vi "Read.vi"(8 "error in (no error)":errorcluster, 11 "Add_WFM in":refnum<class "AbsFunc_Two Term_WFM_Numeric.lvclass">) -> (0 "error out":errorcluster, 2 "Waveform":waveform(dbl), 3 "Add_WFM out":refnum<class "AbsFunc_Two Term_WFM_Numeric.lvclass">)   [LabVIEW 2021, in "AbsFunc_Two Term_WFM_Numeric.lvclass"]
uses:
  AbsFunc_Two Term_WFM_Numeric.lvclass
  AbsFunc_Two Term_WFM_Numeric.lvclass/AbsFunc_Two Term_WFM_Numeric.ctl
  Abs_Types/Waveform/Abs_Waveform.lvclass
  Abs_Types/Numeric/Abs_Numeric.lvclass
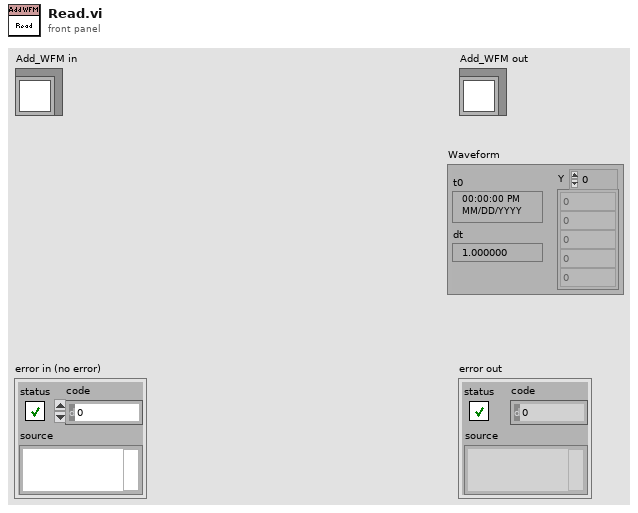
[diagram p1: front panel]
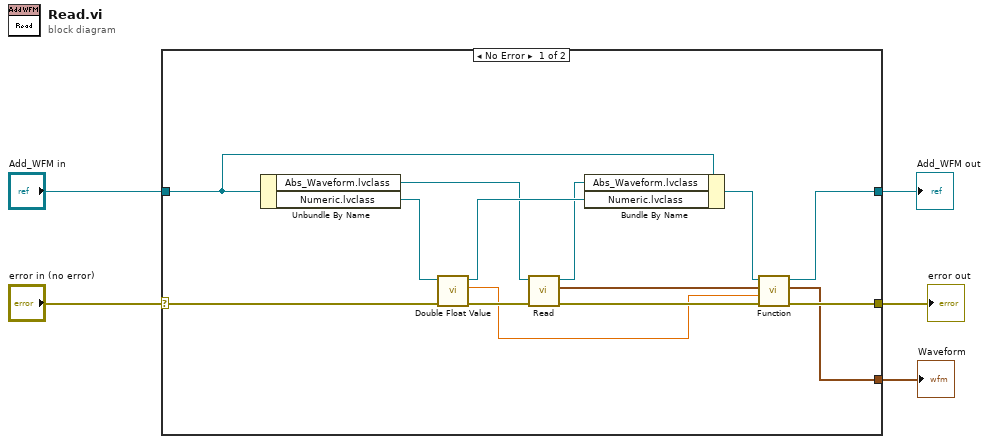
[diagram p0: block diagram]
diagram:
  n1 = case shown="No Error" "error in (no error)" {
    selector: "error in (no error)" -> [w18 w20]
    tunnel: [w19 w20] -> w5
    tunnel: [w16 w21] -> w4
    tunnel: "Add_WFM in" -> [w17 w21]
    tunnel: [w15 _] -> w1
    frame No Error {
      n2 = Unbundle By Name(w17) -> ("Abs_Waveform.lvclass"=w10:refnum<class "Abs_Waveform.lvclass">, "Numeric.lvclass"=w12:refnum<class "Abs_Numeric.lvclass">)
      n3 = call-dynamic "Double Float Value.vi"("error in (no error)"=w18, "Numeric in"=w12) -> ("error out"=w8:errorcluster, "Double"=w6:dbl, "Numeric out"=w11:refnum<class "Abs_Numeric.lvclass">)  [unwired: 7 in]
      n4 = call-dynamic "Read.vi"("error in (no error)"=w8, "Abs_Waveform in"=w10) -> ("error out"=w14:errorcluster, "Waveform"=w7:waveform(dbl), "Abs_Waveform out"=w9:refnum<class "Abs_Waveform.lvclass">)  [unwired: 7 in]
      n5 = Bundle By Name(cluster=w17, "Abs_Waveform.lvclass"=w9, "Numeric.lvclass"=w11) -> (w13:refnum<class "AbsFunc_Two Term_WFM_Numeric.lvclass">)
      n6 = call-dynamic "Function.vi"("error in (no error)"=w14, "Numeric"=w6, "Waveform"=w7, "Two Terminal in"=w13) -> ("error out"=w19:errorcluster, "Result"=w15:waveform(dbl), "Two Terminal out"=w16:refnum<class "AbsFunc_Two Term_WFM_Numeric.lvclass">)  [unwired: 5 in]
    }
    frame Error {
    }
  }
  "error out" <- w5
  "Add_WFM out" <- w4
  "Waveform" <- w1
